vi "libssh2_sftp_write.vi"(8 "error in (no error)":errorcluster, 10 "buffer":string, 11 "sftp handle":T1) -> (0 "error out":errorcluster, 2 "bytes acknowledged":i32)   [LabVIEW 2013, in "libssh2.lvlib"]
doc: "Write data to a file handle."
uses:
  libssh2.lvlib
  SFTP Handle Refnum.ctl
  Not An SFTP Handle Refnum.vi
  <vilib>/Utility/error.llb/Error Cluster From Error Code.vi
  Global Settings.vi
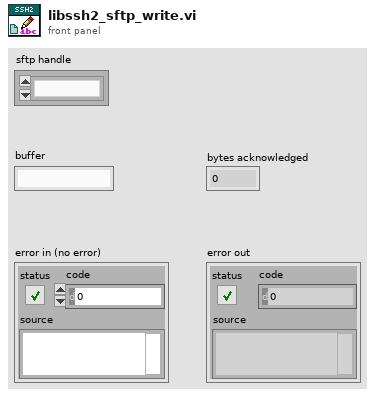
[diagram p1: front panel]
types:
  T1 = typedef "libssh2.lvlib/SFTP Handle Refnum.ctl" = refnum<k1>
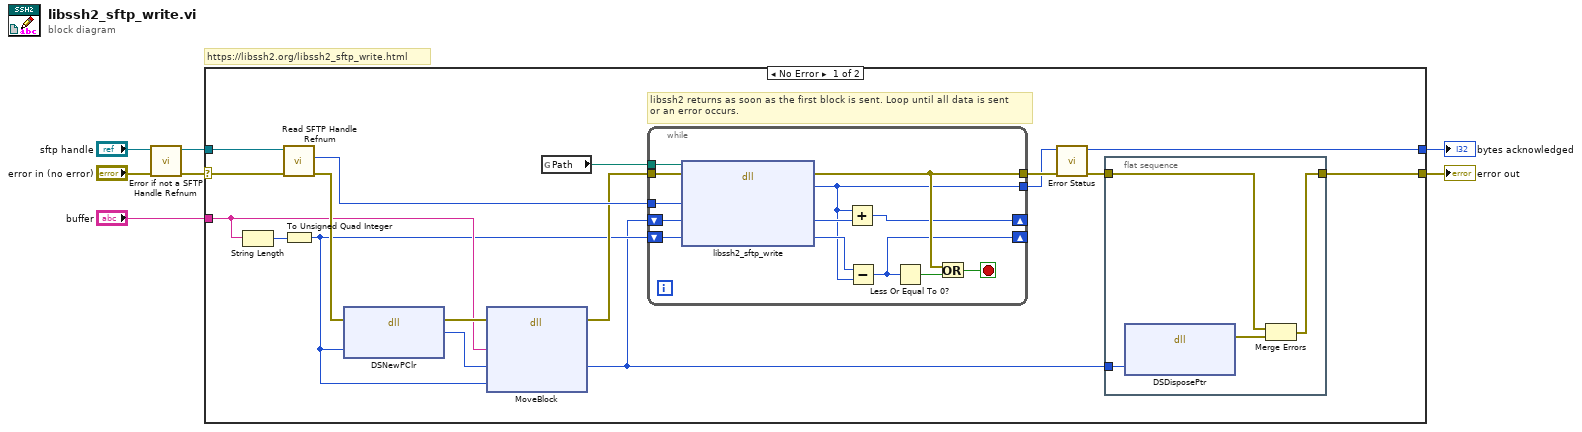
[diagram p0: block diagram]
diagram:
  # "https://libssh2.org/libssh2_sftp_write.html"
  n1 = call "Error if not a SFTP Handle Refnum.vi"("error in (no error)"="error in (no error)", "sftp handle"="sftp handle") -> ("error out"=w6:errorcluster, "sftp handle out"=w5:T1)  [unwired: 8 in]
  n2 = case shown="No Error" w6 {
    selector: w6 -> [w23 w42]
    tunnel: w5 -> [w22 _]
    tunnel: [w13 w42] -> w4
    tunnel: "buffer" -> [w15 _]
    tunnel: [w11 _] -> w1
    frame No Error {
      # "libssh2 returns as soon as the first block is sent. Loop until all data is sent\nor an error occurs."
      n3 = String Length(string=w15) -> (length=w20:i32)
      n4 = call "Read SFTP Handle Refnum.vi"("error in (no error)"=w23, "sftp handle"=w22) -> ("error out"=w17:errorcluster, "LIBSSH2_SFTP_HANDLE*"=w21:u64)  [unwired: 8 in]
      n5 = To Unsigned Quad Integer(1:w20) -> (0:w14:u64)
      n6 = dll-call lib="LabVIEW" fn="DSNewPClr"(error in=w17, "size"=w14) -> (error out=w19:errorcluster, "return type"=w18:u64)  [unwired: 3 in, 1 out]
      n7 = dll-call lib="LabVIEW" fn="MoveBlock"(error in=w19, "ps"=w15, "pd"=w18, "size"=w14) -> (error out=w16:errorcluster, "pd"=w12:u64)  [unwired: 5 in, 1 out]
      n8 = global read "Global Settings.vi" "Path"() -> (w24:path)
      n9 = while {
        tunnel: w24 -> [w37]
        tunnel: w21 -> [w36]
        tunnel: w16 -> [w35]
        tunnel: [w30] -> w9
        shift-right: [w27] -> _
        shift-left: w12 -> [w33]
        shift-right: [w25] -> _
        shift-left: w14 -> [w34]
        tunnel: [w26] -> w8
        stop <- w29 stop-if-true
        n10 = dll-call lib="?" fn="libssh2_sftp_write"(path in=w37, error in=w35, "handle"=w36, "buffer"=w33, "count"=w34) -> (error out=w30:errorcluster, "return value"=w26:i32, "buffer"=w28:u64, "count"=w32:u64)  [unwired: 2 in, 1 out]
        n11 = Add(x=w26, y=w28) -> (x+y=w27:u64)
        n12 = Subtract(x=w32, y=w26) -> (x-y=w25:u64)
        n13 = Less Or Equal To 0?(x=w25) -> (x <= 0?=w31:bool)
        n14 = Or(x=w30, y=w31) -> (x .or. y?=w29:bool)
      }
      n15 = call "Error Status.vi"("error in (no error)"=w9, "return value"=w8) -> ("error out"=w10:errorcluster, "return value out"=w11:i32)  [unwired: 8 in]
      n16 = flat-sequence {
        tunnel: [w39] -> w13
        tunnel: w10 -> [w40]
        tunnel: w12 -> [w41]
        frame #0 {
          n17 = dll-call lib="LabVIEW" fn="DSDisposePtr"("p"=w41) -> (error out=w38:errorcluster)  [unwired: 5 in, 1 out]
          n18 = Merge Errors(w40, w38) -> (w39:errorcluster)
        }
      }
    }
    frame Error {
    }
  }
  "error out" <- w4
  "bytes acknowledged" <- w1
